vi "Get SMO Public API (This Level).vi"(8 "error in (no error)":errorcluster, 11 "Instrument in":refnum<class "Instrument.lvclass">) -> (0 "error out":errorcluster, 2 "commands (this level)":string[](array[string]), 3 "Instrument out":refnum<class "Instrument.lvclass">)   [LabVIEW 2019, in "Instrument.lvclass"]
doc: "Override this VI to return a list of commands only supported by your Instrument"
uses:
  Instrument.lvclass
  Typedefs/Instrument.Commands--Enum.ctl
  a3a974a0-f424-49ae-9768-f4b353ce505d.vi
  <vilib>/Utility/Data Type/Get Numeric Information.vi
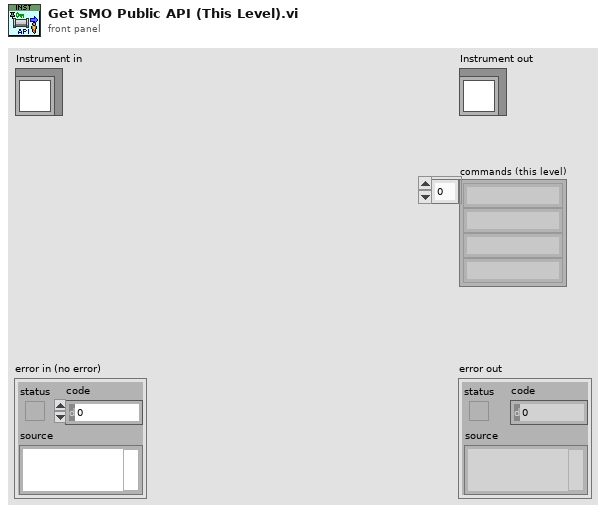
[diagram p1: front panel]
types:
  T1 = typedef "Instrument.lvclass/Instrument.Commands--Enum.ctl" = enum16{"ACK", "HELP", "IDN", "getAll", "getAllData"}
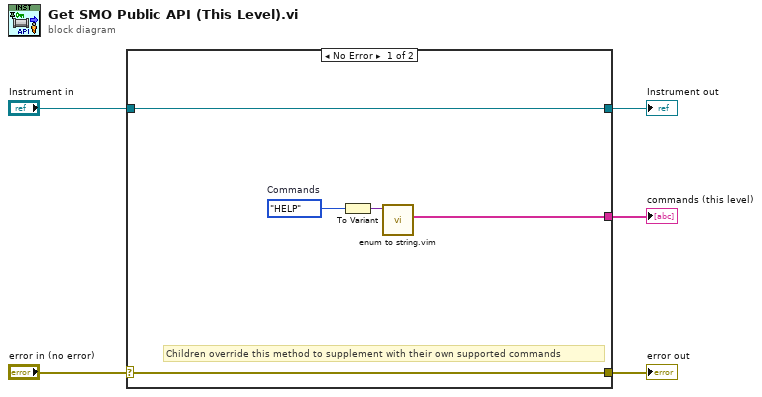
[diagram p0: block diagram]
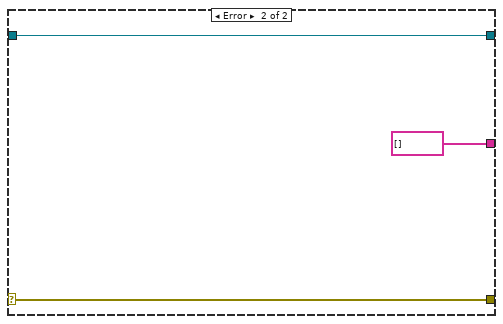
[diagram p2: hidden frame]
diagram:
  n1 = case shown="No Error" "error in (no error)" {
    selector: "error in (no error)" -> [w7 w13]
    tunnel: [w7 w13] -> w4
    tunnel: [w8 w12] -> w2
    tunnel: "Instrument in" -> [w8 w12]
    tunnel: [w9 string[] [] ("Array")] -> w1
    frame No Error {
      w10 = Instrument.Commands--Enum."HELP"  # Commands
      # "Children override this method to supplement with their own supported commands"
      n2 = To Variant(anything=w10) -> (Variant=w6:variant)
      n3 = call "enum to string.vim"("enum in"=w6) -> ("strings out"=w9:string[])  [unwired: 9 in, 1 out]
    }
    frame Error {
    }
  }
  "error out" <- w4
  "Instrument out" <- w2
  "commands (this level)" <- w1
